vi "TA_Split_Data.vi"(11 "Raw TA":dbl[][](array[numeric])=array215x155[33325 elements] format="%#_8g") -> (3 "TA Data":T1)   [LabVIEW 2025]
uses:
  TA_DATA.ctl
panel:
  out "size (raw data)":i32[](array[numeric])
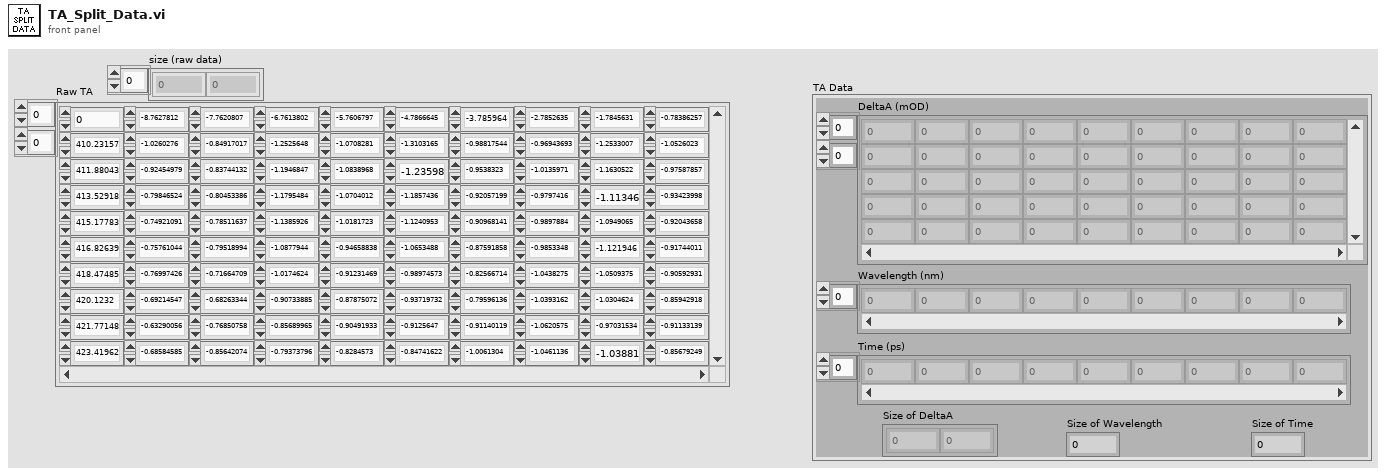
[diagram p1: front panel]
types:
  T1 = typedef "TA_DATA.ctl" = cluster{"DeltaA (mOD)":dbl[][], "Wavelength (nm)":dbl[], "Time (ps)":dbl[], "Size of DeltaA":i32[], "Size of Wavelength":i32, "Size of Time":i32}
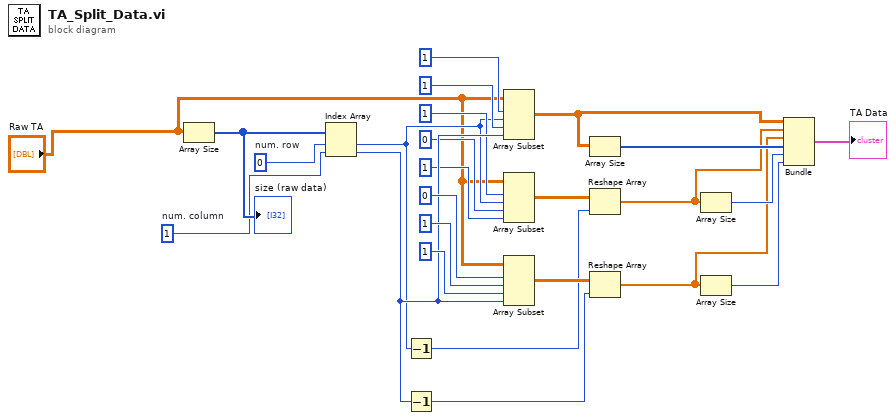
[diagram p0: block diagram]
diagram:
  w18 = 1  # num. column
  w25 = 0  # num. row
  n1 = Array Size(array="Raw TA") -> (size(s)=w22:i32[])
  "size (raw data)" <- w22
  n2 = Index Array "Index Array"(array=w22, index #1=w25, index #2=w18) -> (element #1=w9:i32, element #2=w16:i32)
  n3 = Decrement(x=w9) -> (x-1=w14:i32)
  n4 = Decrement(x=w16) -> (x-1=w15:i32)
  n5 = Array Subset "Array Subset"(array="Raw TA", index (row)=1 ("index"), length (row)=w9, index (col)=1 ("index"), length (col)=w16) -> (w5:dbl[][])
  n6 = Array Subset "Array Subset"(array="Raw TA", index (row)=1 ("index"), length (row)=w9, index (col)=0 ("index"), length (col)=1 ("length")) -> (w13:dbl[][])
  n7 = Array Subset "Array Subset"(array="Raw TA", index (row)=0 ("index"), length (row)=1 ("length"), index (col)=1 ("index"), length (col)=w16) -> (w21:dbl[][])
  n8 = Array Size(array=w5) -> (size(s)=w8:i32[])
  n9 = Reshape Array "Reshape Array"(w13, w14) -> (w4:dbl[])
  n10 = Reshape Array "Reshape Array"(w21, w15) -> (w3:dbl[])
  n11 = Array Size(array=w4) -> (size(s)=w7:i32)
  n12 = Array Size(array=w3) -> (size(s)=w6:i32)
  n13 = Bundle(w5, w4, w3, w8, w7, w6) -> (→"TA Data":cluster{dbl[][], dbl[], dbl[], i32[], i32, i32})  [unwired: 1 in]
